vi "constroi_atp.vi"(1 "archive name":string="teste.atp", 2 "directory out":path=path "C:/ATP/ATPDraw/Projects_Flavio", 5 "dados":string[](array[string]), 9 "Parâmetros":T1, 12 "Frequência":string) -> (4 "concatenated string":string)   [LabVIEW 2020]
panel:
  out "x-y":i32
  in  "Amplitude":dbl=5883.128419 format="%#_10g"
  out "Ger. Distr.":bool
  out "Y / D":bool
  out "Eq. + Trafo":bool
  out "Linhas acopladas":bool
  out "Carga mista":bool
  in  "s":bool=TRUE
  in  "outpus - manual":string="  N0149AN0149BN0149CN0250AN0250BN0250CN0095AN0095BN0095CN0197AN0197BN0197C"
  out "Gd switches":string
  out "Outputs":string
  out "Fault switches":string caption="Result"
  in  "Tab Control":T2(tab)
  out "Mechanical":string="S"
  out "Load (pu)":string="100"
  out "Fault line":string="52_53"
  out "Fault type":string="BCG"
  out "Fault time":string="025"
  out "R fault":string="1"
  out "Event":string
  out "Quantity":string
  out "Node":string
  out "Switches":string
  in  "measure? 3":dbl format="%#_13g"
  out "Lines (atp)":string
  in  "measure?":dbl
  out "Loads (atp)":string
  in  "measure? 2":dbl
  in  "Capacitors (C em uF)":string="  N0083A                   0.001 .0001  36.8                                   0\n  N0083B                   0.001 .0001  36.8                                   0\n  N0083C                   0.001 .0001  36.8                                   0\n  N0088A                   0.001 .0001   9.2                                   0\n  N0090B                   0.001 .0001   9.2                                   0\n  N0092C                   0.001 .0001   9.2                                   0"
  in  "Capacitors (X em uS) - DESLIGADO":string="  N0083A                                36.8                                   0\n  N0083B                                36.8                                   0\n  N0083C                                36.8                                   0\n  N0088A                                 9.2                                   0\n  N0090B                                 9.2                                   0\n  N0092C                                 9.2                                   0"
  in  "Loads":string="spot loads data.csv"
  in  "directory in":path=path "C:/ATP/ATPDraw/Projects_Flavio/feeder123"
  in  "Lines":string="line data.csv"
  in  "Conifgs":string="config.csv"
  in  "Switches 2":string="switch data modif_v2.csv"
  in  "Conifgs (acoplados)":string="config_novo.csv"
  # "1 - current\n2 - voltage\n3 - current e voltage\n4 - power e energy"
  # "ATP Builder - IEEE Test Feeder"
  # "N0149AN0149BN0149CN0013AN0013BN0013CN0018AN0018BN0018CN0250AN0250BN0250CN0151A\n  N0151BN0151CN0095AN0095BN0095CN0060AN0060BN0060CN0197AN0197BN0197C"
  # "N0149AN0149BN0149CN0001AN0001BN0001CN0013AN0013BN0013CN0018AN0018BN0018CN0250A\n  N0250BN0250CN0151AN0151BN0151CN0095AN0095BN0095CN0060AN0060BN0060CN0197AN0197B\n  N0197C"
  # "123 bus IEEE Test Feeder"
  # "valor a direita da virgula E tamanho 6 digitos"
  # "node_node (integers)"
  # "nós:\nde         para"
  # "A                B              C"
  # "A                B              C"
  # "CONFIGURATION"
  # "A"
  # "B"
  # "C"
  # "R     +     X"
  # "R     +     X"
  # "R     +     X"
  # "SWITCHES FAULTS"
  # "S000SAS000NA       -1.      1.E3                                             0\n  S000SBS000NB       -1.      1.E3                                             0\n  S000SCS000NC       -1.      1.E3                                             0\n  S000NAS000OA       -1.      1.E3                                             0\n  S000NBS000OB       -1.      1.E3                                             0\n  S000NCS000OC       -1.      1.E3                                             0\n  S000NAS000ZA      1.E3       -1.                                             0\n  S000NBS000ZB      1.E3       -1.                                             0\n  S000NCS000ZC      1.E3       -1.                                             0\n  S000G             1.E3       -1.                                             0"
  # "N"
  # "nó virtual"
  # "nó da barra"
  # "Z"
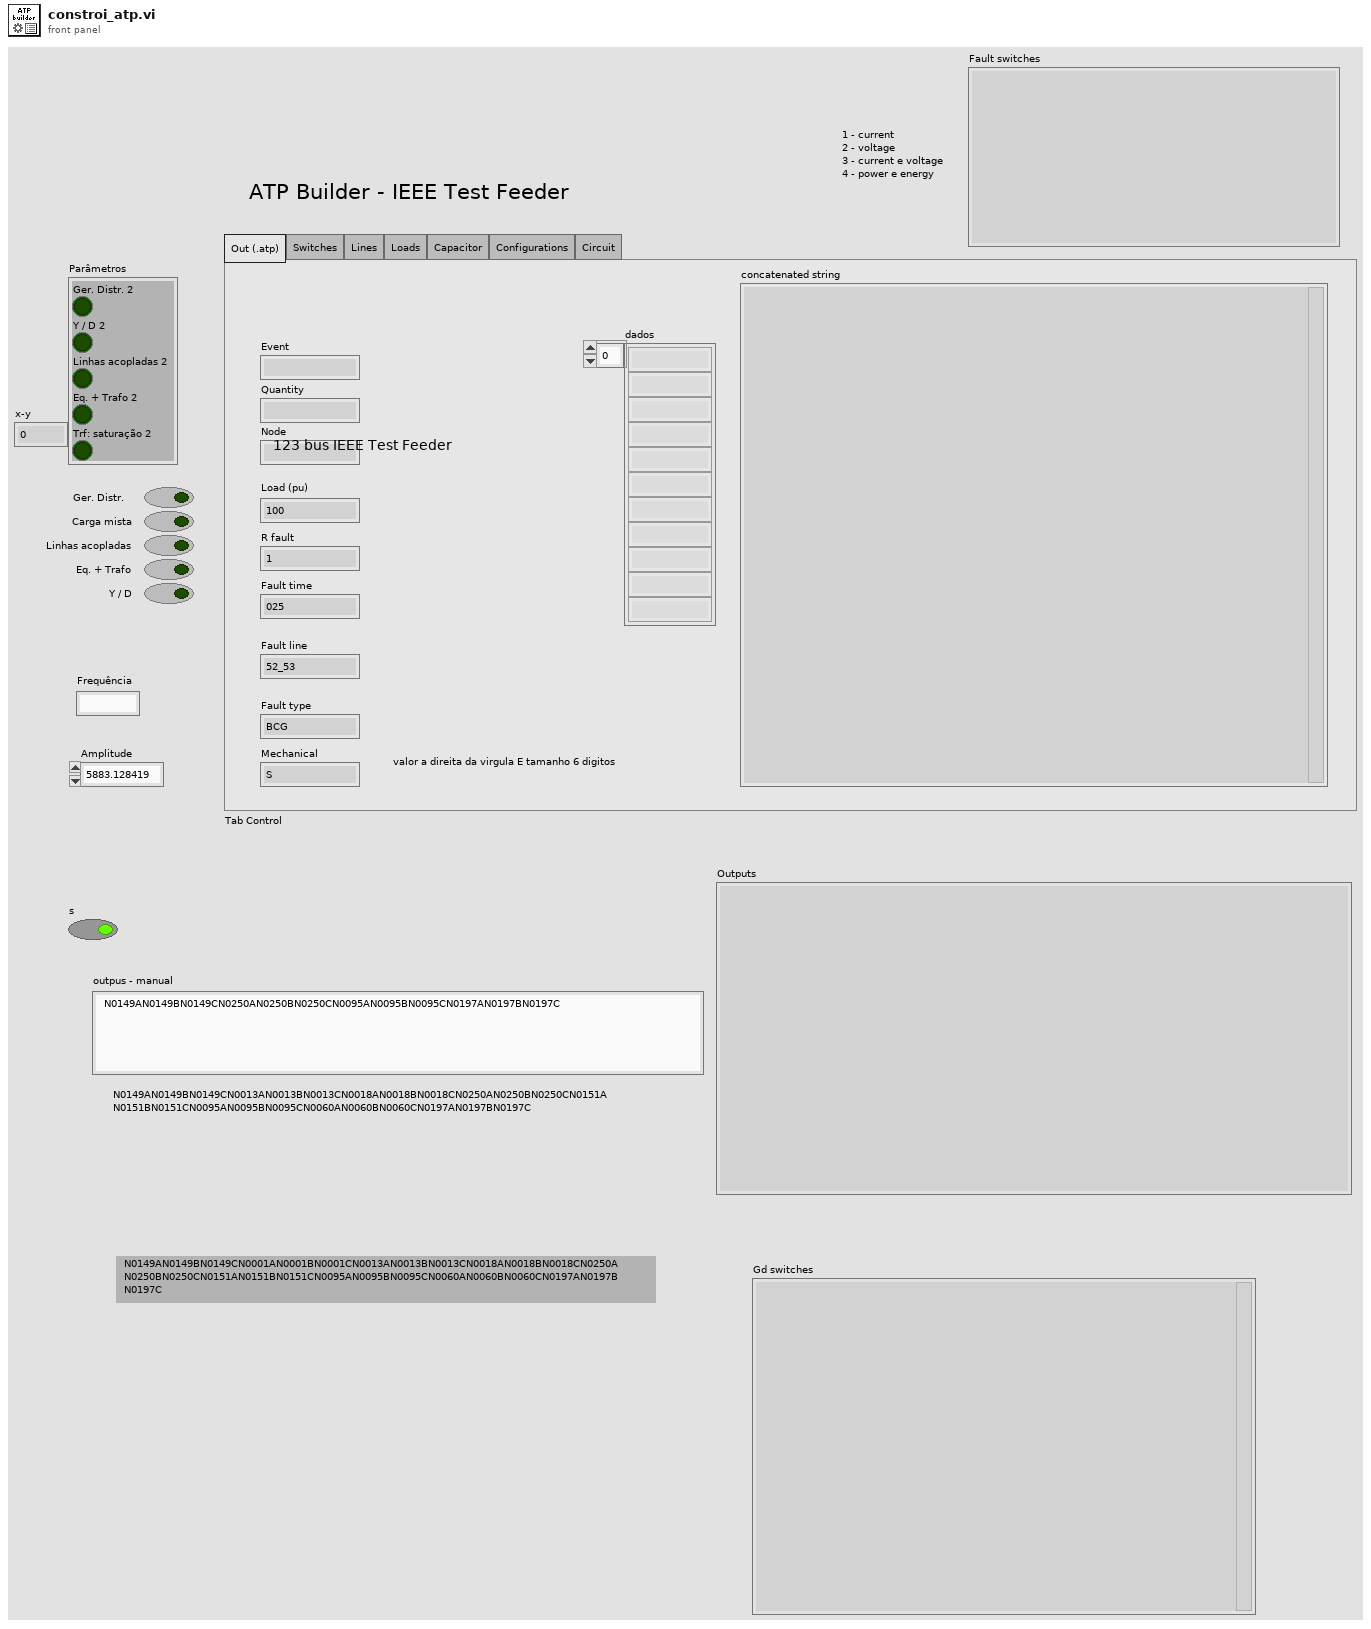
[diagram p1: front panel]
types:
  T1 = cluster{"Ger. Distr. 2":bool, "Y / D 2":bool, "Linhas acopladas 2":bool, "Eq. + Trafo 2":bool, "Trf: saturação 2":bool}
  T2 = enum32{"Out (.atp)", "Switches", "Lines", "Loads", "Capacitor", "Configurations", "Circuit"}
  T3 = enum16{"open", "replace", "create", "open or create", "replace or create", "replace or create with confirmation"}
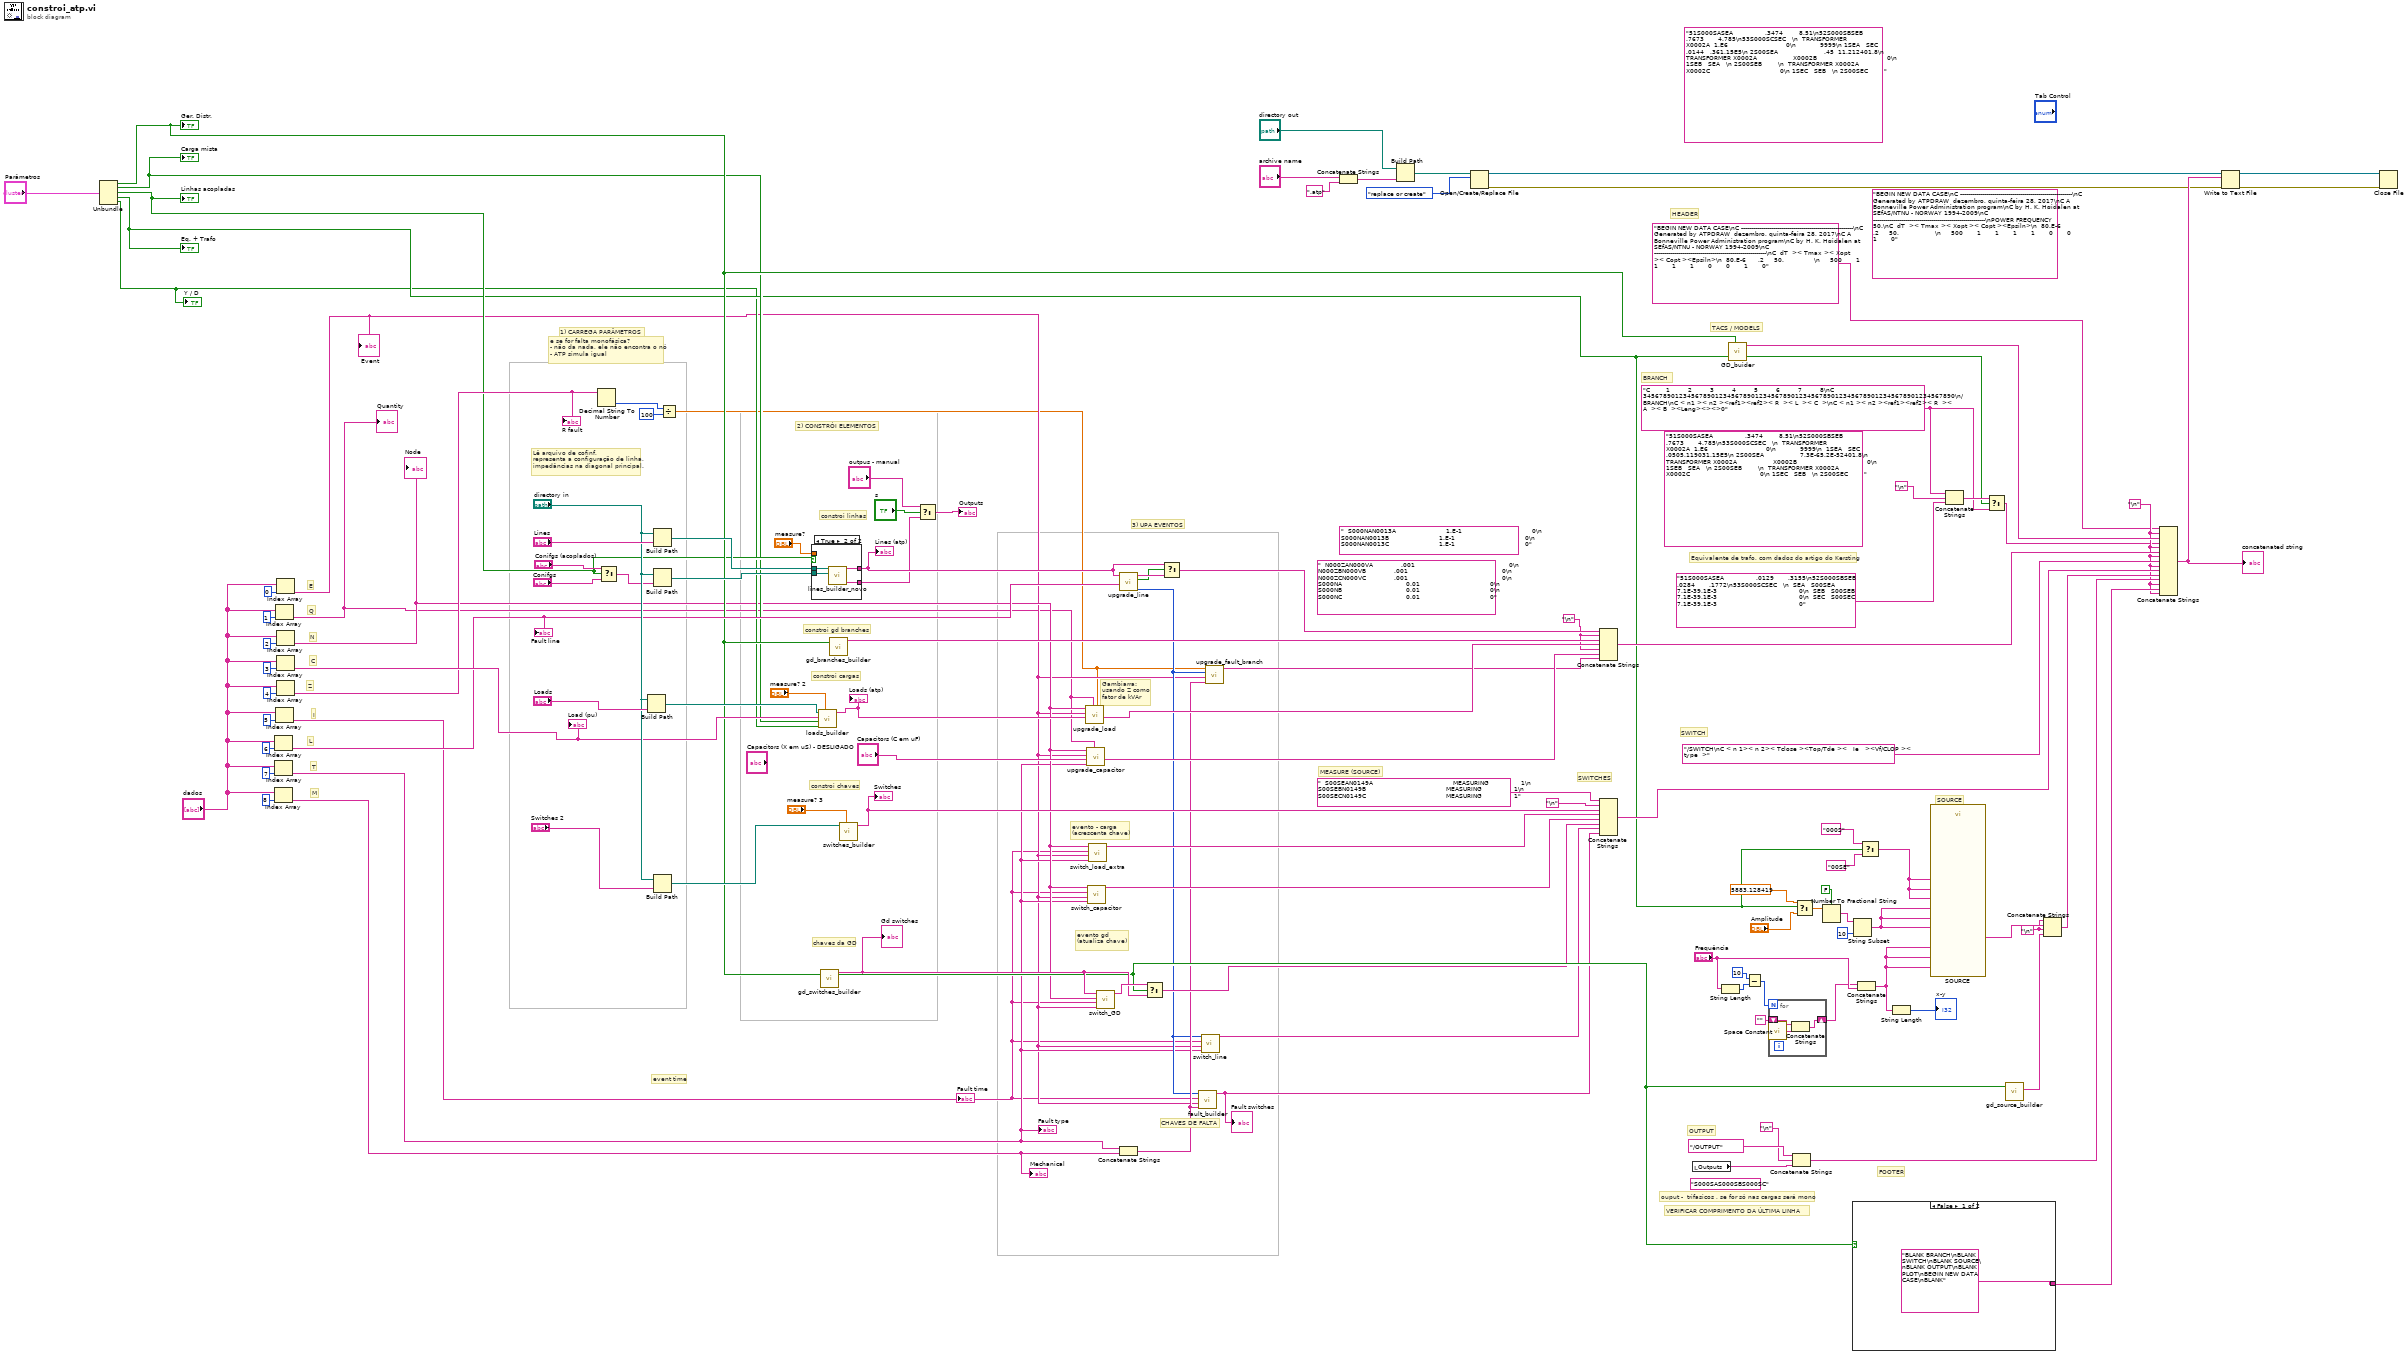
[diagram p0: block diagram]
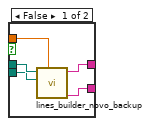
[diagram p2: hidden frame]
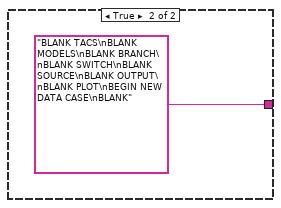
[diagram p3: hidden frame]
diagram:
  (unwired) "  S000NAN0013A                         1.E-1                                   0\n  S000NAN0013B                         1.E-1                                   0\n  S000NAN0013C                         1.E-1                                   0"
  (unwired) "  N000ZAN000VA              .001                                               0\n  N000ZBN000VB              .001                                               0\n  N000ZCN000VC              .001                                               0\n  S000NA                                0.01                                   0\n  S000NB                                0.01                                   0\n  S000NC                                0.01                                   0"
  (unwired) "BEGIN NEW DATA CASE\nC --------------------------------------------------------\nC Generated by ATPDRAW  dezembro, quinta-feira 28, 2017\nC A Bonneville Power Administration program\nC by H. K. Høidalen at SEfAS/NTNU - NORWAY 1994-2009\nC --------------------------------------------------------\nPOWER FREQUENCY                      50.\nC  dT  >< Tmax >< Xopt >< Copt ><Epsiln>\n  80.E-6      .2     50.                  \n     500       1       1       1       1       0       0       1       0"
  (unwired) "51S000SASEA                .3474        8.51\n52S000SBSEB                .7673       4.785\n53S000SCSEC   \n  TRANSFORMER                         X0002A  1.E6                             0\n            9999\n 1SEA   SEC                .0144   .361.15E5\n 2S00SEA                       .45  11.212401.8\n  TRANSFORMER X0002A                  X0002B                                   0\n 1SEB   SEA   \n 2S00SEB        \n  TRANSFORMER X0002A                  X0002C                                   0\n 1SEC   SEB   \n 2S00SEC        "
  (unwired) "51S000SASEA                .3474        8.51\n52S000SBSEB                .7673       4.785\n53S000SCSEC   \n  TRANSFORMER                         X0002A  1.E6                             0\n            9999\n  1SEA   SEC                .0505.119031.15E5\n 2S00SEA                  7.3E-65.2E-52401.8\n  TRANSFORMER X0002A                  X0002B                                   0\n 1SEB   SEA   \n 2S00SEB        \n  TRANSFORMER X0002A                  X0002C                                   0\n 1SEC   SEB   \n 2S00SEC        "
  w22 = "\n"
  (unwired) "S000SAS000SBS000SC"
  w24 = "\n"
  w50 = "\n"
  w42 = "C        1         2         3         4         5         6         7         8\nC 345678901234567890123456789012345678901234567890123456789012345678901234567890\n/BRANCH\nC < n1 >< n2 ><ref1><ref2>< R  >< L  >< C  >\nC < n1 >< n2 ><ref1><ref2>< R  >< A  >< B  ><Leng><><>0"
  # "M"
  # "T"
  # "L"
  # "I"
  # "Z"
  # "C"
  # "N"
  # "Q"
  # "E"
  # "Gambiarra:\nusando Z como\nfator de kVAr"
  # "Equivalente de trafo, com dados do artigo do Kersting"
  # "evento - carga\n(acrescenta chave)"
  # "evento gd\n(atualiza chave)"
  # "chaves da GD"
  # "event time"
  # "constroi gd branches"
  # "TACS / MODELS"
  # "SWITCHES"
  # "ouput -  trifasicos , se for só nas cargas será mono"
  # "1) CARREGA PARÂMETROS"
  # "2) CONSTRÓI ELEMENTOS"
  # "3) UPA EVENTOS"
  # "e se for falta monofásica?\n- não da nada, ele não encontra o nó\n- ATP simula igual"
  # "CHAVES DE FALTA"
  # "VERIFICAR COMPRIMENTO DA ÚLTIMA LINHA"
  # "constroi chaves"
  # "constroi linhas"
  # "constroi cargas"
  # "MEASURE (SOURCE)"
  # "Lê arquivo de cofinf, \nrepresenta a configuração de linha,\nimpedâncias na diagonal principal."
  # "OUTPUT"
  # "FOOTER"
  # "SOURCE"
  # "SWITCH"
  # "BRANCH"
  # "HEADER"
  n1 = Unbundle("Parâmetros") -> ("Ger. Distr. 2"=w46:bool, "Y / D 2"=w38:bool, "Linhas acopladas 2"=w45:bool, "Eq. + Trafo 2"=w29:bool, "Trf: saturação 2"=w28:bool)
  "Carga mista" <- w38
  "Linhas acopladas" <- w45
  "Eq. + Trafo" <- w29
  "Y / D" <- w28
  "Ger. Distr." <- w46
  n2 = Index Array(array="dados", index=8) -> (element=w72:string)
  "Mechanical" <- w72
  n3 = Index Array(array="dados", index=6) -> (element=w75:string)
  "Fault line" <- w75
  n4 = Index Array(array="dados", index=7) -> (element=w14:string)
  "Fault type" <- w14
  n5 = Index Array(array="dados", index=1) -> (element=w10:string)
  "Quantity" <- w10
  n6 = Index Array(array="dados", index=5) -> (element=w12:string)
  "Fault time" <- w12
  n7 = Index Array(array="dados", index=2) -> (element=w19:string)
  "Node" <- w19
  n8 = Index Array(array="dados", index=3) -> (element=w77:string)
  "Load (pu)" <- w77
  n9 = Index Array(array="dados", index=4) -> (element=w76:string)
  "R fault" <- w76
  n10 = Index Array(array="dados", index=0) -> (element=w13:string)
  "Event" <- w13
  n11 = Decimal String To Number(string=w76) -> (number=w62:i32)  [unwired: 2 in, 1 out]
  n12 = Select(t="Conifgs (acoplados)", s=w45, f="Conifgs") -> (s? t:f=w54:string)
  n13 = Build Path(base path="directory in", name or relative path="Loads") -> (appended path=w101:path)
  n14 = Build Path(base path="directory in", name or relative path="Lines") -> (appended path=w105:path)
  n15 = Build Path(base path="directory in", name or relative path=w54) -> (appended path=w104:path)
  n16 = Build Path(base path="directory in", name or relative path="Switches 2") -> (appended path=w99:path)
  n17 = Divide(x=w62, y=100) -> (x/y=w9:dbl)
  n18 = case shown="True" w45 {
    tunnel: w105 -> [w121 w127]
    tunnel: w104 -> [w120 w126]
    tunnel: [w122 w125] -> w94
    tunnel: [w123 w124] -> w61
    tunnel: "measure?" -> [w119 _]
    frame False {
      n19 = call "lines_builder_novo_backup.vi"("measure?"=w119, "Config data"=w120, "Lines data"=w121) -> ("Outputs"=w123:string, "Lines (out)"=w122:string)  [unwired: 5 in, 2 out]
    }
    frame True {
      n20 = call "lines_builder_novo.vi"("Config data"=w126, "Lines data"=w127) -> ("Outputs"=w124:string, "Lines (out)"=w125:string)  [unwired: 6 in, 2 out]
    }
  }
  "Lines (atp)" <- w94
  n21 = call "loads_builder.vi"("measure?"="measure? 2", "D / Y"=w28, "Carga mista"=w38, "Load (%/100)"=w77, "Loads data"=w101) -> ("Loads (out)"=w74:string)  [unwired: 6 in]
  "Loads (atp)" <- w74
  n22 = call "gd_switches_builder.vi"("GD"=w46) -> ("Gd switches"=w64:string)  [unwired: 10 in]
  "Gd switches" <- w64
  n23 = call "gd_branches_builder.vi"("GD"=w46) -> ("GD branches"=w70:string)  [unwired: 10 in]
  n24 = call "switches_builder.vi"("measure?"="measure? 3", "Switches data"=w99) -> ("closed switches (out)"=w95:string)  [unwired: 9 in]
  "Switches" <- w95
  n25 = Select(t="outpus - manual", s="s", f=w61) -> (s? t:f=→"Outputs":string)
  n26 = call "upgrade_load.vi"("fator de kVAr"=w9, "Quantity"=w10, "Loads"=w74, "Event type"=w13, "Node"=w19) -> ("Actual loads"=w69:string)  [unwired: 6 in]
  n27 = call "upgrade_capacitor.vi"("Quantity 2"=w10, "Fault type (phases)"=w14, "Capacitores"="Capacitors (C em uF)", "Event type"=w13, "Node"=w19) -> ("Actual caps"=w49:string)  [unwired: 6 in]
  n28 = call "switch_capacitor.vi"("Node"=w19, "event time"=w12, "Event type"=w13, "Fault type (phases)"=w14) -> ("Event switches"=w20:string)  [unwired: 6 in]
  n29 = call "switch_load_extra.vi"("Node"=w19, "event time"=w12, "Event type"=w13, "Fault type (phases)"=w14) -> ("Event switches"=w18:string)  [unwired: 6 in]
  n30 = call "switch_GD.vi"("Gd switches"=w64, "Node"=w19, "event time"=w12, "Event type"=w13) -> ("updated switch"=w65:string)  [unwired: 6 in]
  n31 = call "upgrade_line.vi"("Lines"=w94, "Fault line"=w75) -> ("Update lines"=w93:string, "ñ encontrado?"=w91:bool, "To"=w15:i32)  [unwired: 4 in, 1 out]
  n32 = Concatenate Strings(w14, w72) -> (w17:string)
  n33 = Select(t=w65, s=w46, f=w64) -> (s? t:f=w23:string)
  n34 = Select(t=w94, s=w91, f=w93) -> (s? t:f=w92:string)
  n35 = call "fault_builder.vi"("Fault type"=w17, "Event type"=w13, "Fault time"=w12, "Node fault"=w15) -> ("Result"=w16:string)  [unwired: 7 in]
  "Fault switches" <- w16
  n36 = call "switch_line.vi"("Node"=w15, "event time"=w12, "Event type"=w13, "Fault type (phases)"=w14) -> ("Event switches"=w11:string)  [unwired: 6 in]
  n37 = call "upgrade_fault_branch.vi"("Fault type"=w17, "Event type"=w13, "node"=w15, "R fault"=w9) -> ("Result"=w21:string)  [unwired: 7 in]
  n38 = Concatenate Strings("archive name", ".atp" ("string")) -> (w88:string)
  n39 = Build Path(base path="directory out", name or relative path=w88) -> (appended path=w108:path)
  n40 = Open/Create/Replace File(file path (use dialog)=w108, operation (0:open)=T3."replace or create") -> (refnum out=w114:refnum<file>, error out=w115:errorcluster)  [unwired: 4 in, 1 out]
  n41 = Concatenate Strings("  S00SEAN0149A                                        MEASURING                1\n  S00SEBN0149B                                        MEASURING                1\n  S00SECN0149C                                        MEASURING                1", "\n", w95, w18, w20, w23, w11, w16) -> (w110:string)
  n42 = Concatenate Strings(w92, w24, w70, w69, w24, w49, w21) -> (w112:string)
  n43 = local read "Outputs"() -> (w67:string)
  n44 = String Length(string="Frequência") -> (length=w8:i32)
  n45 = call "GD_buider.vi"("GD"=w46) -> ("TACS / MODELS"=w71:string)  [unwired: 10 in]
  n46 = Subtract(x=10, y=w8) -> (x-y=w6:i32)
  n47 = for {
    N: w6 -> [_]
    shift-right: [w129] -> w3
    shift-left: "" -> [w128]
    n48 = call <vilib>:"Space Constant.vi"() -> ("String"=w130:string)
    n49 = Concatenate Strings(w128, w130) -> (w129:string)
  }
  n50 = Concatenate Strings("/OUTPUT", "\n", w67) -> (w52:string)
  n51 = Select(t=5883.128419, s=w29, f="Amplitude") -> (s? t:f=w37:dbl)
  n52 = Number To Fractional String(use system decimal point (T)=FALSE, number=w37) -> (F-format string=w39:string)  [unwired: 2 in]
  n53 = case shown="False" w46 {
    tunnel: ["BLANK BRANCH\nBLANK SWITCH\nBLANK SOURCE\nBLANK OUTPUT\nBLANK PLOT\nBEGIN NEW DATA CASE\nBLANK" "BLANK TACS\nBLANK MODELS\nBLANK BRANCH\nBLANK SWITCH\nBLANK SOURCE\nBLANK OUTPUT\nBLANK PLOT\nBEGIN NEW DATA CASE\nBLANK"] -> w51
    frame False {
    }
    frame True {
    }
  }
  n54 = String Subset(string=w39, length (rest)=10 ("length (rest)")) -> (substring=w33:string)  [unwired: 1 in]
  n55 = Concatenate Strings(w3, "Frequência") -> (w2:string)
  n56 = Select(t="000S", s=w29, f="00SE") -> (s? t:f=w30:string)
  n57 = String Length(string=w2) -> (length=→"x-y":i32)
  n58 = call "SOURCE"("nodeA"=w30, "amp_a"=w33, "frequenciaa"=w2, "nodeB"=w30, "amp_b"=w33, "frequenciab"=w2, "nodeC"=w30, "amp_c"=w33, "frequenciac"=w2) -> ("Result"=w34:string)  [unwired: 17 in, 1 out]
  n59 = Concatenate Strings(w42, "\n", "51S000SASEA                .0129       .3155\n52S000SBSEB                .0284       .1772\n53S000SCSEC   \n  SEA   S00SEA            7.1E-39.1E-3                                         0\n  SEB   S00SEB            7.1E-39.1E-3                                         0\n  SEC   S00SEC            7.1E-39.1E-3                                         0") -> (w43:string)
  n60 = Select(t=w43, s=w29, f=w42) -> (s? t:f=w44:string)
  n61 = call "gd_source_builder.vi"("GD"=w46) -> ("Gd switches"=w68:string)  [unwired: 10 in]
  n62 = Concatenate Strings(w22, w34, w22, w68) -> (w53:string)
  n63 = Concatenate Strings("BEGIN NEW DATA CASE\nC --------------------------------------------------------\nC Generated by ATPDRAW  dezembro, quinta-feira 28, 2017\nC A Bonneville Power Administration program\nC by H. K. Høidalen at SEfAS/NTNU - NORWAY 1994-2009\nC --------------------------------------------------------\nC  dT  >< Tmax >< Xopt >< Copt ><Epsiln>\n  80.E-6      .2     50.               \n     500       1       1       1       1       0       0       1       0", w50, w71, w44, w50, w112, w50, "/SWITCH\nC < n 1>< n 2>< Tclose ><Top/Tde ><   Ie   ><Vf/CLOP ><  type  >", w50, w110, w53, w52, w50, w51, w50) -> (w118:string)
  "concatenated string" <- w118
  n64 = Write to Text File(file (use dialog)=w114, text=w118, error in=w115) -> (refnum out=w117:refnum<file>, error out=w116:errorcluster)  [unwired: 1 in, 1 out]
  n65 = Close File(refnum=w117, error in=w116) -> ()  [unwired: 2 out]
